vi "Get and Set Control Disalbe Visible.vi"(8 "错误输入（无错误）":errorcluster, 9 "Mode":enum16{"Read", "Write"}(ring), 10 "Select In":T1, 11 "Ctl Ref In":refnum<vi>) -> (0 "错误输出":errorcluster, 2 "Select Out":T1, 3 "Ctl Ref Out":refnum<vi>)   [LabVIEW 2012, in "CtrlRef.lvlib"]
uses:
  CtrlRef.lvlib
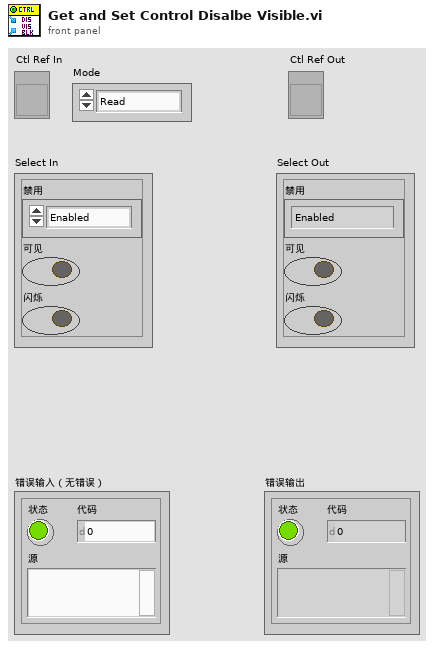
[diagram p1: front panel]
types:
  T1 = cluster{"禁用":enum8{"Enabled", "Disabled", "Disabled and Grayed Out"}, "可见":bool, "闪烁":bool}
  T2 = enum8{"Enabled", "Disabled", "Disabled and Grayed Out"}
  T3 = cluster{"DisabledEnum":enum8{"Enabled", "Disabled", "Disabled and Grayed Out"}, "Visible":bool, "Blinking":bool}
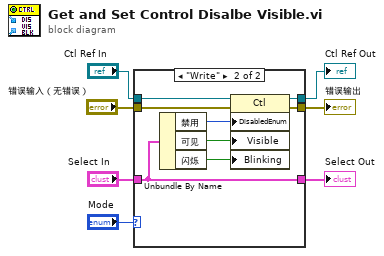
[diagram p0: block diagram]
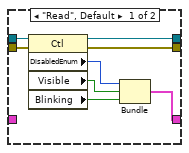
[diagram p2: hidden frame]
diagram:
  n1 = case shown="\"Write\"" "Mode" {
    tunnel: "Select In" -> [_ w22]
    tunnel: [w8 w22] -> w5
    tunnel: "错误输入（无错误）" -> [w14 w19]
    tunnel: [w13 w18] -> w3
    tunnel: "Ctl Ref In" -> [w15 w17]
    tunnel: [w12 w16] -> w1
    frame "Read", Default {
      n2 = property class="Ctl"(reference=w15, error in=w14) -> (reference out=w12:refnum<vi>, error out=w13:errorcluster, "DisabledEnum"=w11:T2, "Visible"=w10:bool, "Blinking"=w9:bool)
      n3 = Bundle("DisabledEnum"=w11, "Visible"=w10, "Blinking"=w9) -> (w8:T3)  [unwired: 1 in]
    }
    frame "Write" {
      n4 = Unbundle By Name(w22) -> ("禁用"=w23:T2, "可见"=w21:bool, "闪烁"=w20:bool)
      n5 = property class="Ctl"(reference=w17, error in=w19, "DisabledEnum"=w23, "Visible"=w21, "Blinking"=w20) -> (reference out=w16:refnum<vi>, error out=w18:errorcluster)
    }
  }
  "错误输出" <- w3
  "Ctl Ref Out" <- w1
  "Select Out" <- w5
